vi "DSF.Engine.Builder.Get ID.vi"(11 "Builder in":refnum<class "DSF.Engine.Builder.lvclass">) -> (2 "ID":i32, 3 "Builder out":refnum<class "DSF.Engine.Builder.lvclass">)   [LabVIEW 2016, in "DSF.Engine.lvlib" / "DSF.Engine.Builder.lvclass"]
uses:
  DSF.Engine.Builder.lvclass
  DSF.Engine.Builder.lvclass/DSF.Engine.Builder.ctl
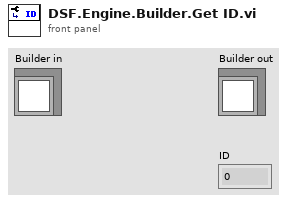
[diagram p1: front panel]
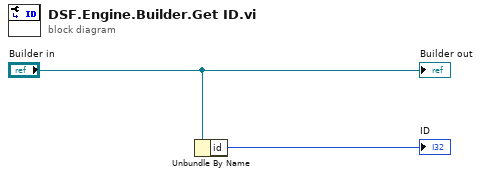
[diagram p0: block diagram]
diagram:
  n1 = Unbundle By Name("Builder in") -> ("id"=→"ID":i32)
  "Builder out" <- "Builder in"
